vi "Load_Source.vi"(8 "error in (no error)":errorcluster, 11 "Installer in":refnum<class "Installer.lvclass">) -> (0 "error out":errorcluster, 3 "Installer out":refnum<class "Installer.lvclass">)   [LabVIEW 2020, in "Installer.lvclass"]
uses:
  <vilib>/AppBuilder/IB_Classes/Installer/Installer.lvclass
  <vilib>/AppBuilder/IB_Classes/Installer/Installer.lvclass/Installer.ctl
  <vilib>/AppBuilder/IB_Classes/Source/IB_Source.lvclass
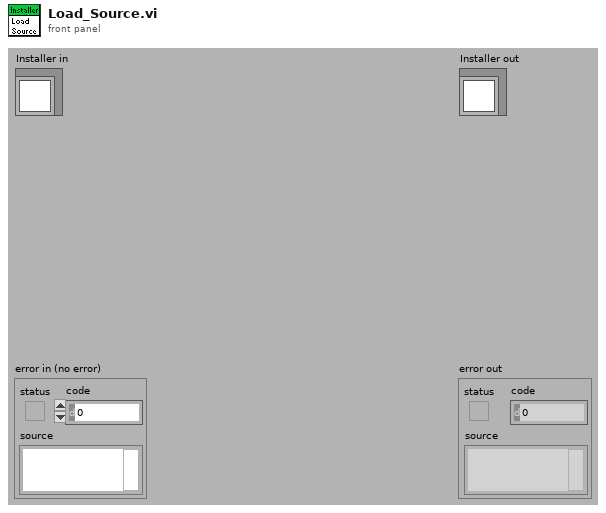
[diagram p1: front panel]
types:
  T1 = typedef "ItemRef.ctl" = u64
  T2 = typedef "IB_Source.ctl" = cluster{"name":string, "sourceTag":string, "destTag":string, "path":path, "eng_installPath":string, "UI_inBuild?":bool, "str ref?":bool}
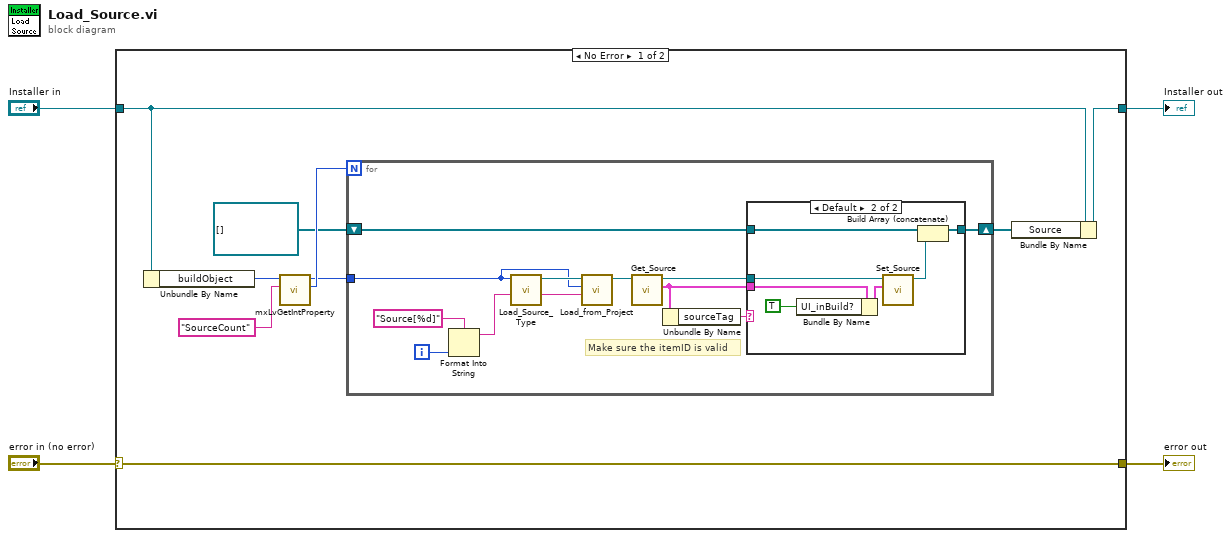
[diagram p0: block diagram]
diagram:
  n1 = case shown="No Error" "error in (no error)" {
    selector: "error in (no error)" -> [w13 w35]
    tunnel: [w13 w35] -> w3
    tunnel: [w5 w34] -> w1
    tunnel: "Installer in" -> [w6 w34]
    frame No Error {
      n2 = Unbundle By Name(w6) -> ("buildObject"=w10:T1)
      n3 = call <resource>:"mxLvGetIntProperty.vi"("Tag"="SourceCount", "Item"=w10) -> ("Value"=w12:i32, "Item"=w11:T1)  [unwired: 7 in, 1 out]
      n4 = for {
        N: w12 -> [_]
        tunnel: w11 -> [w21]
        shift-right: [w25] -> w7
        shift-left: refnum<class "IB_Source.lvclass">[] [] -> [w24]
        i -> [w17]
        # "Make sure the itemID is valid"
        n5 = Format Into String(format string="Source[%d]", w17) -> (resulting string=w16:string)  [unwired: 2 in, 1 out]
        n6 = call <vilib>:"Load_Source_Type.vi"("index in"=w16, "buildObject"=w21) -> ("index out"=w15:string, "IB_Source out"=w22:refnum<class "IB_Source.lvclass">)  [unwired: 7 in, 1 out]
        n7 = call-dynamic "Load_from_Project.vi"("index in"=w15, "buildObject"=w21, "IB_Source in"=w22) -> ("IB_Source out"=w20:refnum<class "IB_Source.lvclass">)  [unwired: 5 in, 3 out]
        n8 = call <vilib>:"Get_Source.vi"("IB_Source in"=w20) -> ("data"=w14:T2, "IB_Source out"=w19:refnum<class "IB_Source.lvclass">)  [unwired: 8 in, 1 out]
        n9 = Unbundle By Name(w14) -> ("sourceTag"=w23:string)
        n10 = case shown="Default" w23 {
          tunnel: w19 -> [_ w31]
          tunnel: [w26 w33] -> w25
          tunnel: w24 -> [w26 w32]
          tunnel: w14 -> [_ w29]
          frame "" {
          }
          frame Default {
            n11 = Bundle By Name(cluster=w29, "UI_inBuild?"=TRUE) -> (w28:T2)
            n12 = call <vilib>:"Set_Source.vi"("data"=w28, "IB_Source in"=w31) -> ("IB_Source out"=w30:refnum<class "IB_Source.lvclass">)  [unwired: 8 in, 1 out]
            n13 = Build Array (concatenate)(w32, w30) -> (w33:refnum<class "IB_Source.lvclass">[])
          }
        }
      }
      n14 = Bundle By Name(cluster=w6, "Source"=w7) -> (w5:refnum<class "Installer.lvclass">)
    }
    frame Error {
    }
  }
  "error out" <- w3
  "Installer out" <- w1
